vi "Time Message Events.vi"(8 "error in (no error)":errorcluster, 9 "Debug Mode":bool, 10 "Message in":T1={"Command"="", "Data"=variant(string ""), "ID"="", "error"={"status"=FALSE, "code"=0, "source"=""}}, 11 "RemoteControl":refnum<class "RemoteControl.lvclass">) -> (0 "error out":errorcluster, 1 "time (ms)":u32, 2 "Message out":T1={"Command"="", "Data"=variant(string ""), "ID"="", "error"={"status"=FALSE, "code"=0, "source"=""}}, 3 "RemoteControl out":refnum<class "RemoteControl.lvclass">)   [LabVIEW 2019, in "RemoteControl.lvlib" / "RemoteControl.lvclass"]
uses:
  RemoteControl.lvclass
  Typedefs/Message--Cluster.ctl
  <vilib>/Utility/Data Type/Type Definitions/Data Type.ctl
  <vilib>/Utility/Data Type/NI_Data Type.lvlib
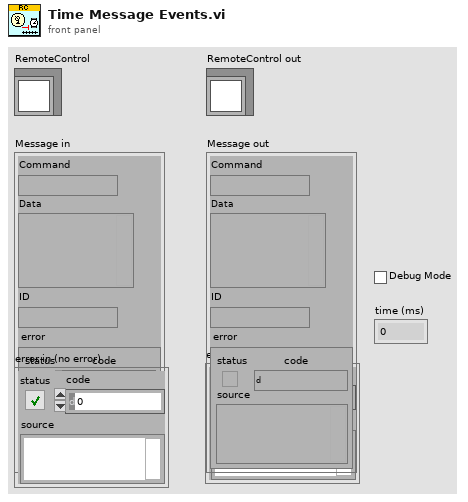
[diagram p1: front panel]
types:
  T1 = typedef "RemoteControl.lvlib/RemoteControl.lvclass/Message--Cluster.ctl" = cluster{"Command":string, "Data":variant, "ID":string, "error":errorcluster}
  T2 = typedef "NI_Data Type.lvlib/Data Type.ctl" = enum8{"Invalid Type", "Void", "I8", "I16", "I32", "I64", "U8", "U16", "U32", "U64", "Single Float", "Double Float", "Extended Float", "Single Complex", "Double Complex", "Extended Complex", "Enum U8", "Enum U16", "Enum U32", "Enum U64", "Single Float With Unit", "Double Float With Unit", "Extended Float With Unit", "Single Complex with Unit", "Double Complex with Unit", "Extended Complex with Unit", "Boolean", "String", "Path", "Picture", "Tag", "Array", "Cluster", "Variant", "LV Variant", "Waveform", "Timestamp", "Digital Waveform", "Digital Data", "ExpressData", "Refnum", "External Data", "VI", "Poly VI", "LabVIEW Class Instance", "Fixed Point", "Set Collection", "Map Collection"}
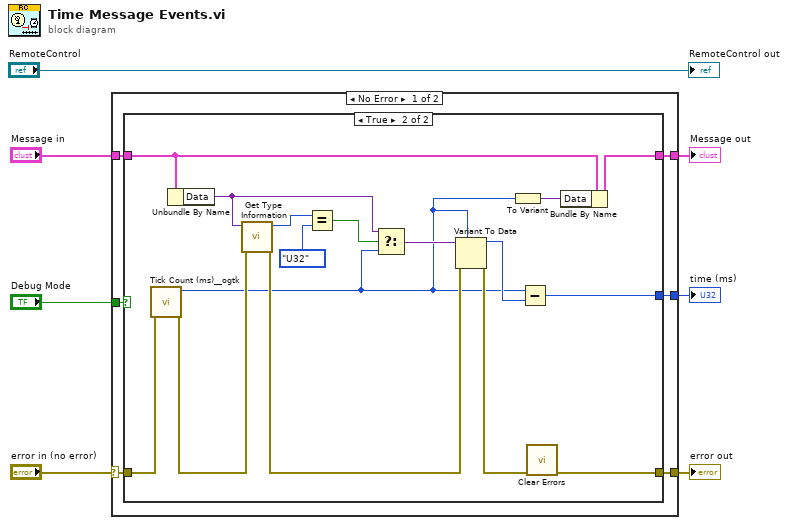
[diagram p0: block diagram]
diagram:
  n1 = case shown="No Error" "error in (no error)" {
    selector: "error in (no error)" -> [w8 w33]
    tunnel: [w13 w33] -> w7
    tunnel: [w12 _] -> w6
    tunnel: [w11 w32] -> w5
    tunnel: "Message in" -> [w10 w32]
    tunnel: "Debug Mode" -> [w9 _]
    frame No Error {
      n2 = case shown="True" w9 {
        tunnel: [w14 w24] -> w13
        tunnel: w8 -> [w14 w29]
        tunnel: [_ w28] -> w12
        tunnel: [w15 w27] -> w11
        tunnel: w10 -> [w15 w26]
        frame False {
        }
        frame True {
          n3 = call <userlib>:"Tick Count (ms)__ogtk.vi"("error in (no error)"=w29) -> ("error out"=w23:errorcluster, "millisecond timer value"=w16:u32)  [unwired: 9 in]
          n4 = Unbundle By Name(w26) -> ("Data"=w19:variant)
          n5 = call <vilib>:"Get Type Information.vi"("error in (no error)"=w23, "variant"=w19) -> ("error out"=w22:errorcluster, "type"=w20:T2)  [unwired: 5 in, 3 out]
          n6 = Equal?(x=w20, y=Data_Type."U32" ("Type")) -> (x = y?=w18:bool)
          n7 = Select(t=w19, s=w18, f=w16) -> (s? t:f=w17:variant)
          n8 = Variant To Data(error in=w22, type=w16, Variant=w17) -> (data=w31:u32, error out=w30:errorcluster)
          n9 = To Variant(anything=w16) -> (Variant=w25:variant)
          n10 = Subtract(x=w16, y=w31) -> (x-y=w28:u32)
          n11 = call <vilib>:"Clear Errors.vi"("error in (no error)"=w30) -> ("error out"=w24:errorcluster)  [unwired: 5 in, 1 out]
          n12 = Bundle By Name(cluster=w26, "Data"=w25) -> (w27:T1)
        }
      }
    }
    frame Error {
    }
  }
  "error out" <- w7
  "Message out" <- w5
  "time (ms)" <- w6
  "RemoteControl out" <- "RemoteControl"
